vi "LC_Relay_Definite Time.vi"(2 "transfer in":bool, 4 "transfer trip in":bool, 6 "instantaneous reset after tripping? (F)":bool, 7 "timing values in":T3, 8 "trip signal in":bool, 9 "time delay settings":T1, 10 "pick-up signal? (F)":bool, 11 "status in":T2) -> (0 "transfer trip out":bool, 1 "trip signal out":bool, 3 "status out":T2, 5 "timing values out":T3)   [LabVIEW 2016]
doc: "Outputs trip decision based on definite time settings."
uses:
  <vilib>/addons/Electrical Power/Protection/Definite Time Delay/subVIs/fpga_Timer Feedback Var.ctl
  <vilib>/addons/Electrical Power/Protection/Definite Time Delay/subVIs/fpga_State.ctl
  <vilib>/addons/Electrical Power/Protection/Definite Time Delay/subVIs/fpga_Time Delay Cfg.ctl
  <vilib>/addons/Electrical Power/Protection/NI_EP_Protection_FPGA.lvlib
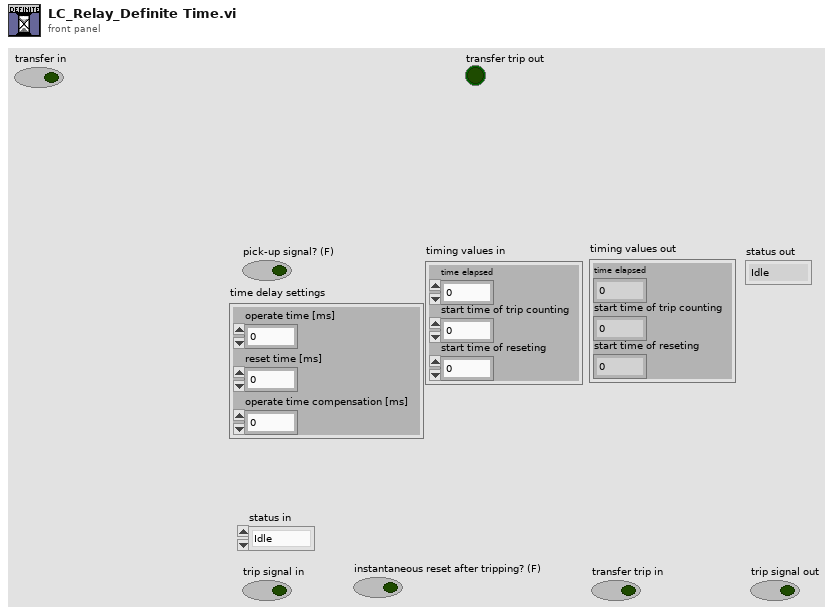
[diagram p1: front panel]
types:
  T1 = typedef "NI_EP_Protection_FPGA.lvlib/fpga_Time Delay Cfg.ctl" = cluster{"operate time [ms]":u32, "reset time [ms]":u32, "operate time compensation [ms]":u32}
  T2 = typedef "NI_EP_Protection_FPGA.lvlib/fpga_State.ctl" = enum16{"Idle", "Trip Counting", "Tripped", "Reset Counting"}
  T3 = typedef "NI_EP_Protection_FPGA.lvlib/fpga_Timer Feedback Var.ctl" = cluster{"time elapsed":u32, "start time of trip counting":u32, "start time of reseting":u32}
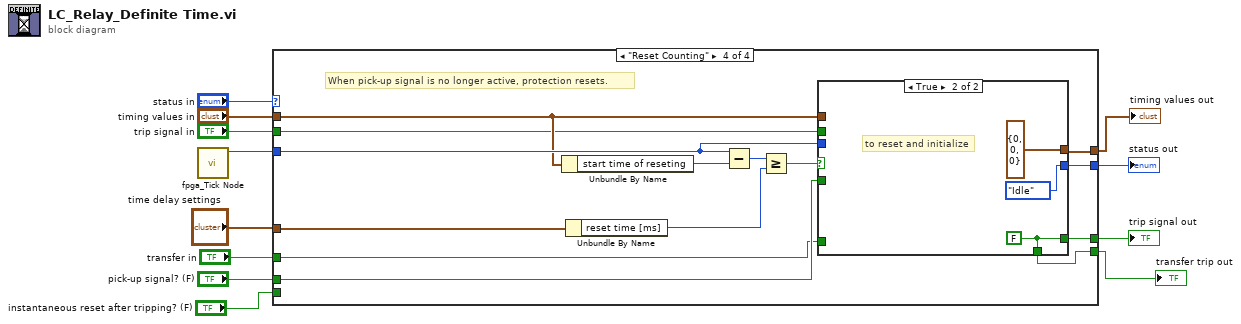
[diagram p0: block diagram]
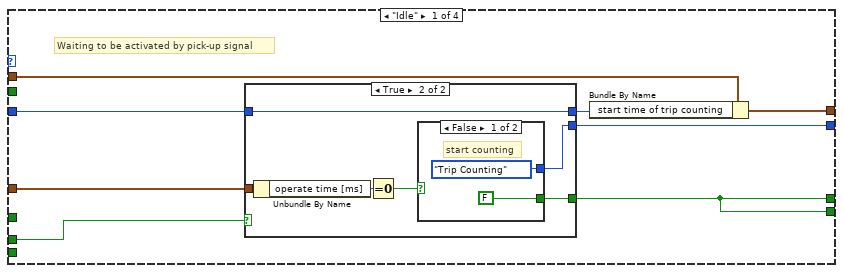
[diagram p2: hidden frame]
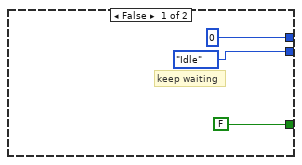
[diagram p3: hidden frame]
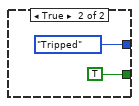
[diagram p4: hidden frame]
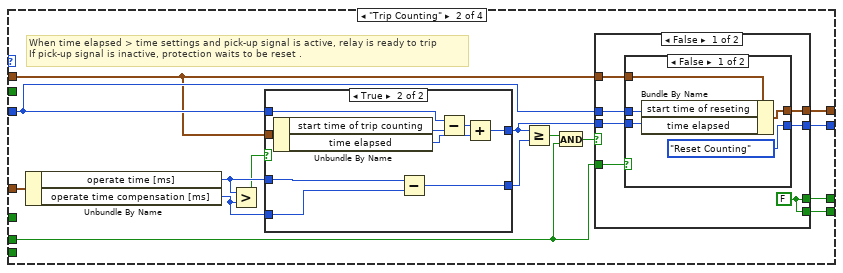
[diagram p5: hidden frame]
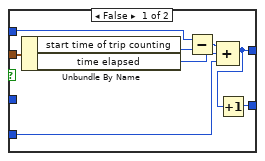
[diagram p6: hidden frame]
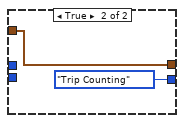
[diagram p7: hidden frame]
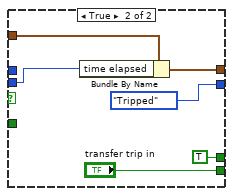
[diagram p8: hidden frame]
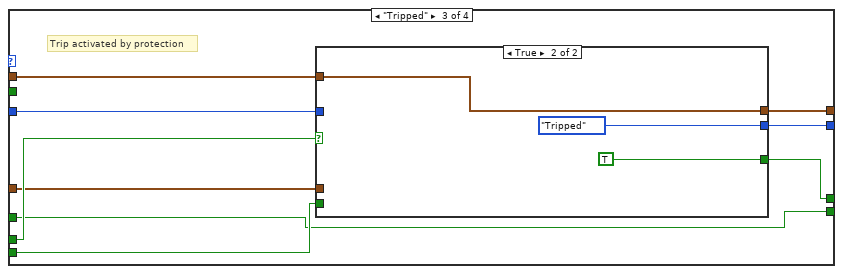
[diagram p9: hidden frame]
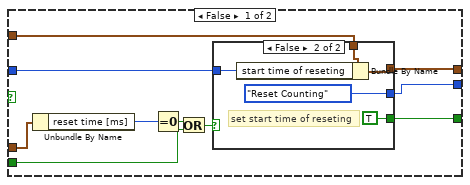
[diagram p10: hidden frame]
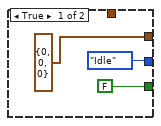
[diagram p11: hidden frame]
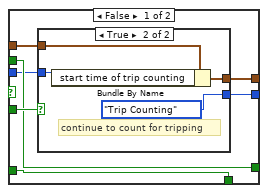
[diagram p12: hidden frame]
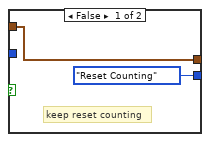
[diagram p13: hidden frame]
diagram:
  n1 = call <vilib>:"fpga_Tick Node.vi"() -> ("millisecond timer value"=w5:u32)  [unwired: 11 in]
  n2 = case shown="\"Reset Counting\"" "status in" {
    tunnel: "pick-up signal? (F)" -> [w20 w43 w94 w120]
    tunnel: [w17 w48 w92 w127] -> w9
    tunnel: [w13 w47 w89 w128] -> w7
    tunnel: "trip signal in" -> [_ _ _ w119]
    tunnel: "timing values in" -> [w18 w35 w91 w124]
    tunnel: [w19 w40 w90 w123] -> w10
    tunnel: w5 -> [w16 w42 w93 w125]
    tunnel: "time delay settings" -> [w14 w39 w88 w122]
    tunnel: "instantaneous reset after tripping? (F)" -> [_ _ w87 _]
    tunnel: [w13 w34 w86 w117] -> w2
    tunnel: "transfer in" -> [_ _ w86 w116]
    frame "Idle" {
      # "Waiting to be activated by pick-up signal"
      n3 = case shown="True" w20 {
        tunnel: [fpga_State."Idle" w24] -> w17
        tunnel: w16 -> [_ w29]
        tunnel: [u32 0 ("Tick Count(mSec)") w29] -> w15
        tunnel: w14 -> [_ w27]
        tunnel: [FALSE ("trip?") w25] -> w13
        frame False {
          # "keep waiting"
        }
        frame True {
          n4 = Unbundle By Name(w27) -> ("operate time [ms]"=w28:u32)
          n5 = Equal To 0?(x=w28) -> (x = 0?=w26:bool)
          n6 = case shown="False" w26 {
            tunnel: [FALSE ("trip?") TRUE ("trip?")] -> w25
            tunnel: [fpga_State."Trip Counting" fpga_State."Tripped"] -> w24
            frame False {
              # "start counting"
            }
            frame True {
            }
          }
        }
      }
      n7 = Bundle By Name(cluster=w18, "start time of trip counting"=w15) -> (w19:T3)
    }
    frame "Trip Counting" {
      # "When time elapsed > time settings and pick-up signal is active, relay is ready to trip\nIf pick-up signal is inactive, protection waits to be reset ."
      n8 = Unbundle By Name(w39) -> ("operate time [ms]"=w38:u32, "operate time compensation [ms]"=w37:u32)
      n9 = Greater?(x=w38, y=w37) -> (0:w36:bool)
      n10 = case shown="True" w36 {
        tunnel: [w50 w64] -> w44
        tunnel: w42 -> [w53 w63]
        tunnel: [w51 w61] -> w41
        tunnel: w38 -> [_ w59]
        tunnel: w37 -> [w52 w58]
        tunnel: w35 -> [w49 w60]
        frame False {
          n11 = Unbundle By Name(w49) -> ("start time of trip counting"=w55:u32, "time elapsed"=w54:u32)
          n12 = Subtract(x=w53, y=w55) -> (x-y=w56:u32)
          n13 = Compound Arithmetic op=ADD(w56, w54, w52) -> (w50:u32)
          n14 = Increment(x=w50) -> (x+1=w51:u32)
        }
        frame True {
          n15 = Unbundle By Name(w60) -> ("start time of trip counting"=w62:u32, "time elapsed"=w57:u32)
          n16 = Subtract(x=w59, y=w58) -> (x-y=w61:u32)
          n17 = Subtract(x=w63, y=w62) -> (x-y=w65:u32)
          n18 = Add(x=w65, y=w57) -> (x+y=w64:u32)
        }
      }
      n19 = Greater Or Equal?(x=w44, y=w41) -> (x >= y?=w45:bool)
      n20 = And(x=w45, y=w43) -> (x .and. y?=w46:bool)
      n21 = case shown="False" w46 {
        tunnel: [w71 fpga_State."Tripped"] -> w48
        tunnel: [w66 TRUE ("trip?")] -> w47
        tunnel: w43 -> [w72 _]
        tunnel: w44 -> [w70 w81]
        tunnel: w42 -> [w69 _]
        tunnel: [w68 w82] -> w40
        tunnel: w35 -> [w67 w83]
        tunnel: [w66 "transfer trip in"] -> w34
        frame False {
          w66 = FALSE ("trip?")
          n22 = case shown="False" w72 {
            tunnel: [fpga_State."Reset Counting" fpga_State."Trip Counting"] -> w71
            tunnel: w70 -> [w75 _]
            tunnel: w69 -> [w76 _]
            tunnel: [w74 w78] -> w68
            tunnel: w67 -> [w73 w78]
            frame False {
              n23 = Bundle By Name(cluster=w73, "start time of reseting"=w76, "time elapsed"=w75) -> (w74:T3)
            }
            frame True {
            }
          }
        }
        frame True {
          n24 = Bundle By Name(cluster=w83, "time elapsed"=w81) -> (w82:T3)
        }
      }
    }
    frame "Tripped" {
      # "Trip activated by protection"
      n25 = case shown="True" w94 {
        tunnel: [w104 fpga_State."Tripped"] -> w92
        tunnel: w93 -> [w101 _]
        tunnel: w91 -> [w102 w114]
        tunnel: [w103 w114] -> w90
        tunnel: [w100 TRUE ("trip?")] -> w89
        tunnel: w88 -> [w98 _]
        tunnel: w87 -> [w96 _]
        frame False {
          n26 = Unbundle By Name(w98) -> ("reset time [ms]"=w99:u32)
          n27 = Equal To 0?(x=w99) -> (x = 0?=w97:bool)
          n28 = Or(x=w97, y=w96) -> (x .or. y?=w95:bool)
          n29 = case shown="False" w95 {
            tunnel: [fpga_State."Idle" fpga_State."Reset Counting"] -> w104
            tunnel: [T3 {"time elapsed"=0, "start time of trip counting"=0, "start time of reseting"=0} ("timer in") w111] -> w103
            tunnel: w102 -> [_ w110]
            tunnel: w101 -> [_ w109]
            tunnel: [FALSE TRUE] -> w100
            frame True {
            }
            frame False {
              # "set start time of reseting"
              n30 = Bundle By Name(cluster=w110, "start time of reseting"=w109) -> (w111:T3)
            }
          }
        }
        frame True {
        }
      }
    }
    frame "Reset Counting" {
      # "When pick-up signal is no longer active, protection resets."
      n31 = Unbundle By Name(w124) -> ("start time of reseting"=w126:u32)
      n32 = Unbundle By Name(w122) -> ("reset time [ms]"=w121:u32)
      n33 = Subtract(x=w125, y=w126) -> (x-y=w129:u32)
      n34 = Greater Or Equal?(x=w129, y=w121) -> (x >= y?=w118:bool)
      n35 = case shown="True" w118 {
        tunnel: [w134 w143] -> w128
        tunnel: w119 -> [w134 _]
        tunnel: [w135 fpga_State."Idle"] -> w127
        tunnel: w120 -> [w136 _]
        tunnel: w125 -> [w133 _]
        tunnel: w124 -> [w132 _]
        tunnel: [w131 T3 {"time elapsed"=0, "start time of trip counting"=0, "start time of reseting"=0} ("timer in")] -> w123
        tunnel: [w130 w143] -> w117
        tunnel: w116 -> [w130 _]
        frame False {
          n36 = case shown="True" w136 {
            tunnel: [fpga_State."Reset Counting" fpga_State."Trip Counting"] -> w135
            tunnel: w133 -> [_ w142]
            tunnel: w132 -> [w137 w141]
            tunnel: [w137 w140] -> w131
            frame False {
              # "keep reset counting"
            }
            frame True {
              # "continue to count for tripping"
              n37 = Bundle By Name(cluster=w141, "start time of trip counting"=w142) -> (w140:T3)
            }
          }
        }
        frame True {
          w143 = FALSE ("trip?")
          # "to reset and initialize"
        }
      }
    }
  }
  "timing values out" <- w10
  "status out" <- w9
  "trip signal out" <- w7
  "transfer trip out" <- w2
